vi "Wrapper_Create.vi"() -> (0 "Wrapper":u32)   [LabVIEW 2017]
uses:
  OmniDriver32.dll
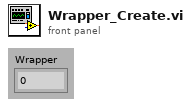
[diagram p1: front panel]
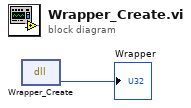
[diagram p0: block diagram]
diagram:
  n1 = dll-call lib="OmniDriver32.dll" fn="Wrapper_Create" label="Wrapper.Create"() -> (→"Wrapper":u32)  [unwired: 3 in, 2 out]
